vi "Write All Gain and Phase.vi"(8 "error in (no error)":errorcluster, 10 "All Gain and Phase":cluster{"Gain":dbl, "Phase":dbl}[](array[cluster]), 11 "Sinusoidal Fit in":refnum<class "Sinusoidal Fit.lvclass">) -> (0 "error out":errorcluster, 3 "Sinusoidal Fit out":refnum<class "Sinusoidal Fit.lvclass">)   [LabVIEW 2016, in "Sinusoidal Fit.lvclass"]
uses:
  Sinusoidal Fit.lvclass
  Sinusoidal Fit.lvclass/Sinusoidal Fit.ctl
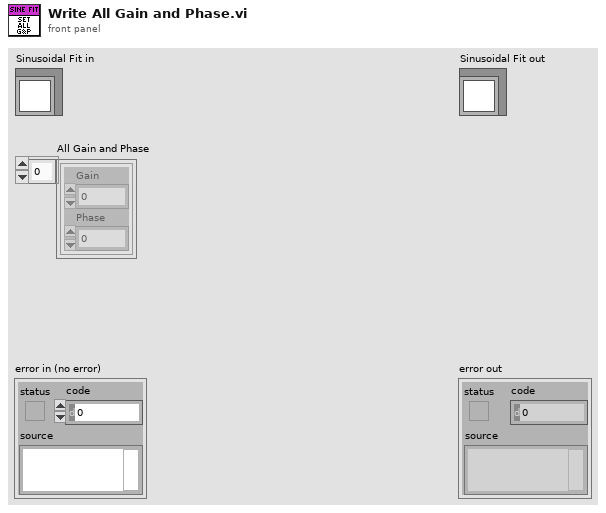
[diagram p1: front panel]
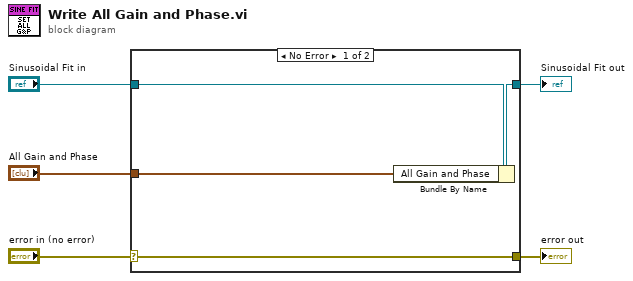
[diagram p0: block diagram]
diagram:
  n1 = case shown="No Error" "error in (no error)" {
    selector: "error in (no error)" -> [w9 w10]
    tunnel: [w9 w10] -> w4
    tunnel: [w7 w11] -> w2
    tunnel: "Sinusoidal Fit in" -> [w8 w11]
    tunnel: "All Gain and Phase" -> [w6 _]
    frame No Error {
      n2 = Bundle By Name(cluster=w8, "All Gain and Phase"=w6) -> (w7:refnum<class "Sinusoidal Fit.lvclass">)
    }
    frame Error {
    }
  }
  "error out" <- w4
  "Sinusoidal Fit out" <- w2
